vi "Master(상태머신).vi"() -> ()   [LabVIEW 2014]
panel:
  out "에러 출력":errorcluster
  out "열거형":T1(ring)
  in  "정지":bool
  out "웨이브폼 그래프":dbl[](graph)
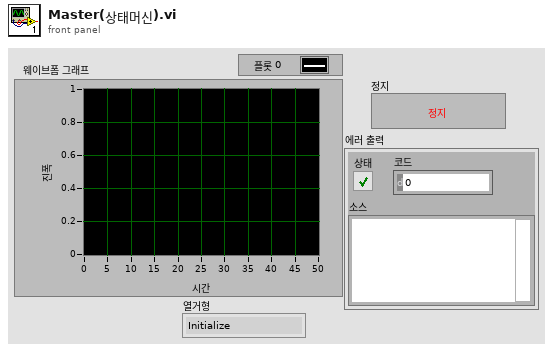
[diagram p1: front panel]
types:
  T1 = enum16{"Initialize", "Wait Connection", "Communication", "Stop"}
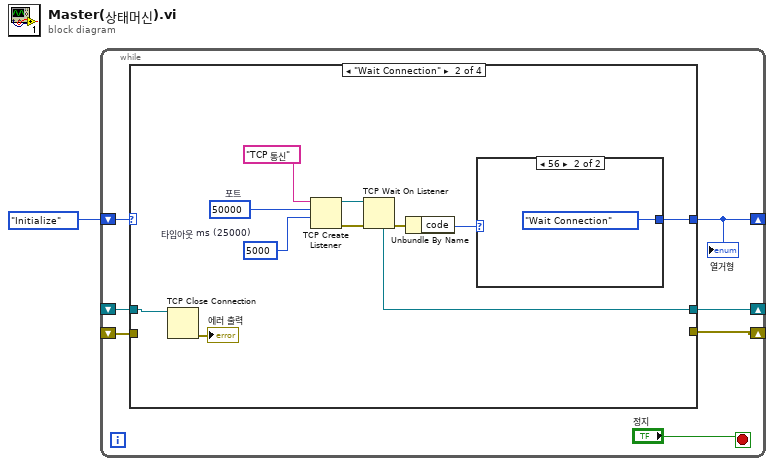
[diagram p0: block diagram]
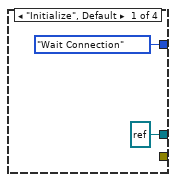
[diagram p2: hidden frame]
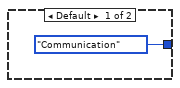
[diagram p3: hidden frame]
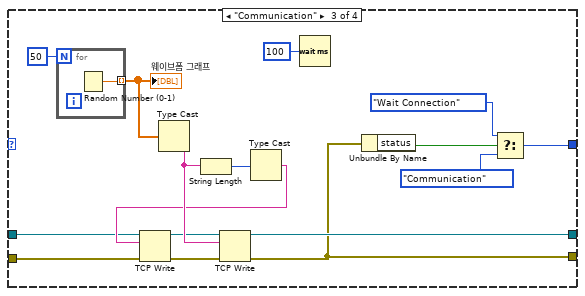
[diagram p4: hidden frame]
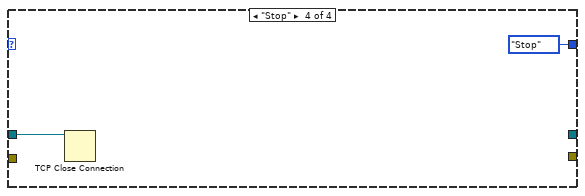
[diagram p5: hidden frame]
diagram:
  n1 = while {
    shift-right: [w7] -> _
    shift-left: T1."Initialize" ("열거형") -> [w8]
    shift-right: [w6] -> _
    shift-left: _ -> [w5]
    shift-right: [w3] -> _
    shift-left: _ -> [w2]
    stop <- "정지" stop-if-true
    n2 = case shown="\"Wait Connection\"" w8 {
      tunnel: [T1."Wait Connection" ("열거형") w15 w31 T1."Stop" ("열거형")] -> w7
      tunnel: [refnum<k5> refnum ("listener ID") w14 w29 _] -> w6
      tunnel: w5 -> [_ w12 w32 w41]
      tunnel: [_ _ w25 _] -> w3
      tunnel: w2 -> [_ _ w26 _]
      frame "Initialize", Default {
      }
      frame "Wait Connection" {
        w21 = 5000  # 타임아웃 ms (25000)
        w20 = u16 50000  # 포트
        n3 = TCP Close Connection(connection ID=w12) -> (error out=→"에러 출력":errorcluster)  [unwired: 2 in, 1 out]
        n4 = TCP Create Listener(9:w21, 10:w20, 11:"TCP 통신" ("서비스 이름")) -> (0:w17:errorcluster, 3:w18:refnum<k5>)  [unwired: 2 in, 1 out]
        n5 = TCP Wait On Listener(8:w17, 11:w18) -> (0:w13:errorcluster, 4:w14:refnum<k5>)  [unwired: 2 in, 3 out]
        n6 = Unbundle By Name(w13) -> ("code"=w16:i32)
        n7 = case shown="56" w16 {
          tunnel: [T1."Communication" ("열거형") T1."Wait Connection" ("열거형")] -> w15
          frame Default {
          }
          frame 56 {
          }
        }
      }
      frame "Communication" {
        n8 = for {
          N: 50 -> [_]
          tunnel: [w40] -> w35 mode=indexing
          n9 = Random Number (0-1)() -> (number: 0 to 1=w40:dbl)
        }
        "웨이브폼 그래프" <- w35
        n10 = Type Cast(x=w35) -> (*(type *) &x=w39:string)  [unwired: 1 in]
        n11 = String Length(string=w39) -> (length=w36:i32)
        n12 = Type Cast(x=w36) -> (*(type *) &x=w38:string)  [unwired: 1 in]
        n13 = TCP Write(connection ID=w32, data in=w38, error in (no error)=w26) -> (connection ID out=w33:refnum<k5>, error out=w37:errorcluster)  [unwired: 1 in, 1 out]
        n14 = TCP Write(connection ID=w33, data in=w39, error in (no error)=w37) -> (connection ID out=w29:refnum<k5>, error out=w25:errorcluster)  [unwired: 1 in, 1 out]
        n15 = Wait (ms)(milliseconds to wait=u32 100 ("대기 시간(ms)")) -> ()  [unwired: 1 out]
        n16 = Unbundle By Name(w25) -> ("status"=w24:bool)
        n17 = Select(t=T1."Wait Connection" ("열거형"), s=w24, f=T1."Communication") -> (s? t:f=w31:T1)
      }
      frame "Stop" {
        n18 = TCP Close Connection(connection ID=w41) -> ()  [unwired: 2 in, 2 out]
      }
    }
    "열거형" <- w7
  }
